vi "BCU参数读取-Auto.vi"(8 "CAN端口":u16(ring), 9 "设备索引号":u16(ring), 10 "CAN卡类型":u32(ring)=21, 11 "Myindex":dbl=1.0) -> (3 "成功":bool)   [LabVIEW 2013] (continued)
      n15 = property on="SOC(%)" class="DigNum (严格)"("Disabled"=w39) -> ()  [unwired: 2 in, 2 out]
      n16 = local write "等级 2"(T19."从板信息" ("等级 2")) -> ()
      n17 = local write "主板2"(T8."项目信息" ("主从板")) -> ()
      n18 = property class="MCListbox (严格)"(reference=w44, "ItemNames"=w40) -> ()  [unwired: 1 in, 2 out]
      n19 = property class="MCListbox (严格)"(reference=w43, "ItemNames"=w40) -> ()  [unwired: 1 in, 2 out]
      n20 = property class="MCListbox (严格)"(reference=w42, "ItemNames"=w40) -> ()  [unwired: 1 in, 2 out]
      n21 = property class="Bool (严格)"(reference=w61, "BoolText.TextColor"=u32 87470) -> ()  [unwired: 1 in, 2 out]
      n22 = property class="Bool (严格)"(reference=w62, "BoolText.TextColor"=w36) -> ()  [unwired: 1 in, 2 out]
      n23 = local write "主从板"(enum32{"单选选项2", "单选选项1"}."单选选项1" ("主从板")) -> ()
      n24 = property on="项目信息2" class="Clust (严格)"("DisabledEnum"=w39) -> ()  [unwired: 2 in, 2 out]
      n25 = property on="系统时钟" class="Str"("Disabled"=w39) -> ()  [unwired: 2 in, 2 out]
      n26 = property on="配置文件版本" class="Str"("Disabled"=w39) -> ()  [unwired: 2 in, 2 out]
      n27 = property on="车架(牌)号" class="Str"("Disabled"=w39) -> ()  [unwired: 2 in, 2 out]
      n28 = property on="产品编号" class="Str"("Disabled"=w39) -> ()  [unwired: 2 in, 2 out]
      n29 = property on="从板号" class="DigNum (严格)"("NumText.BGColor"=w36) -> ()  [unwired: 2 in, 2 out]
      n30 = property on="单选选项2 2" class="Bool (严格)"("BoolText.TextColor"=w36) -> ()  [unwired: 2 in, 2 out]
      n31 = local write "面板选择"(T7."读写参数" ("面板选择")) -> ()
      n32 = property on="单选选项1" class="Bool (严格)"("BoolText.TextColor"=u32 5898201) -> ()  [unwired: 2 in, 2 out]
      n33 = property on="单选选项2" class="Bool (严格)"("BoolText.TextColor"=w36) -> ()  [unwired: 2 in, 2 out]
      n34 = local write "主界面选项"(enum32{"单选选项1", "单选选项2", "单选选项2 2", "单选选项2 3"}."单选选项1" ("主界面选项")) -> ()
      n35 = local write "判定3"(w46) -> ()
      n36 = local write "清BUFF"(w46) -> ()
      n37 = local write "1"(w46) -> ()
      n38 = property on="从板个数" class="DigNum (严格)"("Visible"=w46) -> ()  [unwired: 2 in, 2 out]
      n39 = property on="从板个数" class="DigNum (严格)"("NumText.BGColor"=u32 16448250) -> ()  [unwired: 2 in, 2 out]
      n40 = Not(x=w46) -> (.not. x?=w65:bool)
      n41 = property on="主板选项" class="Tree (严格)"("Visible"=w46) -> ()  [unwired: 2 in, 2 out]
      n42 = property on="全部写入" class="Bool (严格)"("DisabledEnum"=2) -> ()  [unwired: 2 in, 2 out]
      n43 = property on="当前从板板号" class="DigNum (严格)"("Visible"=w65) -> ()  [unwired: 2 in, 2 out]
      n44 = property on="从板选项" class="Tree (严格)"("Visible"=w65) -> ()  [unwired: 2 in, 2 out]
      n45 = control-ref of="结果"() -> (w52:refnum<vi>)
      n46 = control-ref of="结果"() -> (w49:refnum<vi>)
      n47 = local write "强制停止版本读取"(w38) -> ()
      n48 = local write "强制终止读写标记"(w38) -> ()
      n49 = control-ref of="项目信息"() -> (w50:refnum<vi>)
      n50 = local write "判定2"(w38) -> ()
      n51 = local write "停止"(w38) -> ()
      n52 = local write "控制1"(w38) -> ()
      n53 = local write "消除"(w38) -> ()
      n54 = global write "EV05全局变量1.vi" "授权功能"(w38) -> ()
      n55 = local write "继电器超时处理"(w38) -> ()
      n56 = local write "1 6"(w38) -> ()
      n57 = local write "1 7"(w38) -> ()
      n58 = local write "1 8"(w38) -> ()
      n59 = local write "1 9"(w38) -> ()
      n60 = local write "1 10"(w38) -> ()
      n61 = local write "1 2"(w38) -> ()
      n62 = local write "1 3"(w38) -> ()
      n63 = local write "1 4"(w38) -> ()
      n64 = local write "1 5"(w38) -> ()
      n65 = local write "1 11"(w38) -> ()
      n66 = for {
        N: 100 -> [_]
        tunnel: w52 -> [w88]
        i -> [w86]
        n67 = Bundle(w86, 0) -> (w84:cluster{i32, i32})  [unwired: 1 out]
        n68 = property class="MCListbox (严格)"(reference=w88, "ActiveCell"=w84, "CellBG"=u32 16448250) -> ()  [unwired: 1 in, 2 out]
      }
      n69 = for {
        N: 100 -> [_]
        tunnel: w50 -> [w83]
        i -> [w82]
        n70 = Bundle(w82, 0) -> (w80:cluster{i32, i32})  [unwired: 1 out]
        n71 = property class="Tbl (严格)"(reference=w83, "Active Cell"=w80, "Cell BG Color"=u32 16448250) -> ()  [unwired: 1 in, 2 out]
      }
      n72 = for {
        N: 100 -> [_]
        tunnel: w49 -> [w93]
        i -> [w91]
        n73 = Bundle(w91, 0) -> (w89:cluster{i32, i32})  [unwired: 1 out]
        n74 = property class="MCListbox (严格)"(reference=w93, "ActiveCell"=w89, "CellBG"=u32 16448250) -> ()  [unwired: 1 in, 2 out]
      }
      n75 = stacked-sequence {
        tunnel: [_ w67] -> w45
        frame #0 {
          w66 = u32 21 items=["PCI5121"=1, "PCI9810"=2, "USBCAN1"=3, "USBCAN2"=4, "PCI9820"=5, "PCI5110"=7, "CANLite(mini)"=8, "ISA9620"=9, "ISA5420"=10, "PC104CAN"=11, "DNP9810"=13, "PCI9840B"=14, "PC104C2"=15, "PCI9820I"=16, "pec9920"=18, "USBCAN_E_U"=20, "USBCAN_2E_U"=21] ("CAN卡类型")
          n76 = local write "CAN卡类型"(w66) -> ()
        }
        frame #1 {
          w74 = u8 0 items=["Normal", "Listen Only"] ("工作方式")
          w73 = u8 1 items=["Dual Filter", "Single Filter"] ("滤波方式")
          n77 = local read "CAN卡类型"() -> (w68:u32)
          n78 = local read "设备索引号"() -> (w69:u16)
          n79 = local read "CAN端口"() -> (w70:u16)
          n80 = call "CAN_Init-8.6.vi"("CAN卡类型"=w68, "设备索引号"=w69, "CAN端口"=w70, "操作类型"=enum16{"初始化CAN", "关闭CAN"}."初始化CAN", "滤波方式"=w73, "Accept Code"=u32 3221225472, "簇"=T21 {"打开CAN"=TRUE, "初始化CAN"=TRUE, "开始CAN"=TRUE, "重启"=FALSE, "关闭CAN"=FALSE}, "Mask Code"=u32 1073741823 ("Accept Code"), "工作方式"=w74, "是否滤波"=TRUE, "滤波选择"=T20 {"fiter_mode"=1, "fiter_endid"=402653184, "fiter_startid"=419430399}) -> ("error out"=w67:errorcluster)  [unwired: 3 in, 5 out]
        }
      }
      n81 = local write "加热继电器(从)"(w38) -> ()
      n82 = local write "风机继电器(从)"(w38) -> ()
      n83 = local write "DO1"(w38) -> ()
      n84 = local write "DO2"(w38) -> ()
      n85 = local write "DO1 2"(w38) -> ()
      n86 = local write "正级继电器"(w38) -> ()
      n87 = local write "负级继电器"(w38) -> ()
      n88 = local write "加热继电器"(w38) -> ()
      n89 = local write "充电继电器"(w38) -> ()
      n90 = local write "风机继电器"(w38) -> ()
      n91 = local write "预充电继电器"(w38) -> ()
      n92 = property on="保存版本信息" class="Bool (严格)"("Visible"=w38) -> ()  [unwired: 2 in, 2 out]
      n93 = property on="单个读取" class="Bool (严格)"("Visible"=w38) -> ()  [unwired: 2 in, 2 out]
      n94 = property on="单个写入" class="Bool (严格)"("Visible"=w38) -> ()  [unwired: 2 in, 2 out]
      n95 = local write "正级继电器 12"(w38) -> ()
      n96 = local write "正级继电器 2"(w38) -> ()
      n97 = local write "正级继电器 3"(w38) -> ()
      n98 = local write "正级继电器 4"(w38) -> ()
      n99 = local write "正级继电器 5"(w38) -> ()
      n100 = local write "正级继电器 6"(w38) -> ()
      n101 = local write "正级继电器 7"(w38) -> ()
      n102 = local write "正级继电器 8"(w38) -> ()
      n103 = local write "正级继电器 9"(w38) -> ()
      n104 = local write "正级继电器 10"(w38) -> ()
      n105 = local write "正级继电器 11"(w38) -> ()
      n106 = property on="从板号" class="DigNum (严格)"("Visible"=w38) -> ()  [unwired: 2 in, 2 out]
      "电池故障" <- w40
      "模块版本值" <- w57
      "硬件版本" <- w58
      "模块版本名称" <- w57
      "平台软件版本" <- w58
      "项目软件版本" <- w58
      "模块个数" <- u8[] [0, 0, 0, 0, 0, 0, 0, 0, 0, 0, 0, 0, 0, 0, 0, 0, 0, 0, 0, 0, 0, 0, 0, 0, 0, 0, 0, 0, 0, 0, 0, 0] ("模块个数")
    }
  }
  n107 = stacked-sequence {
    tunnel: [w94] -> w24
    frame #0 {
      n108 = call <vilib>:"Set Busy.vi"() -> ()  [unwired: 10 in, 2 out]
      n109 = disable-structure shown="禁用" {
        frame Disabled {
          n110 = control-ref of="主板选项"() -> (w213:refnum<vi>)
          n111 = stacked-sequence {
            tunnel: w213 -> [w215 w373 w411]
            frame #0 {
              # "加热和充电控制参数"
              n112 = global read "功能码全局.vi" "主板控制类信息10"() -> (w225:bool[])
              n113 = Index Array(array=w225) -> (element #5=w219:bool, element #6=w217:bool, element #7=w218:bool, element #8=w216:bool)  [unwired: 8 in, 4 out]
              n114 = Not Or(1:w218, 2:w219) -> (0:w224:bool)
              n115 = Not Or(1:w216, 2:w217) -> (0:w222:bool)
              n116 = for {
                N: 8 -> [_]
                tunnel: w215 -> [w345]
                tunnel: w224 -> [w341]
                tunnel: [w340] -> w223
                i -> [w343]
                n117 = Add(x=w343, y=69) -> (x+y=w344:i32)
                n118 = property class="Tree (严格)"(reference=w345, "Active Item Row Number"=w344, "Disabled?"=w341) -> (error out=w340:errorcluster)  [unwired: 1 in, 1 out]
              }
              n119 = for {
                N: 9 -> [_]
                tunnel: w215 -> [w339]
                tunnel: w222 -> [w335]
                tunnel: w223 -> [w334]
                tunnel: [w333] -> w214
                i -> [w337]
                n120 = Add(x=w337, y=77) -> (x+y=w338:i32)
                n121 = property class="Tree (严格)"(reference=w339, error in=w334, "Active Item Row Number"=w338, "Disabled?"=w335) -> (error out=w333:errorcluster)  [unwired: 1 out]
              }
              n122 = stacked-sequence {
                tunnel: w215 -> [w245 _ _]
                tunnel: w214 -> [w244 _ _]
                frame #0 {
                  # "电池信息"
                  n123 = global read "功能码全局.vi" "主板版本号11"() -> (w246:bool[])
                  n124 = global read "功能码全局.vi" "主板项目信息4"() -> (w228:bool[])
                  n125 = Index Array(array=w246) -> (element #1=w242:bool, element #2=w241:bool, element #3=w235:bool, element #4=w229:bool, element #6=w234:bool, element #7=w233:bool, element #8=w232:bool)  [unwired: 8 in, 1 out]
                  n126 = Index Array(array=w228, index=4 ("索引")) -> (element=w226:bool)
                  n127 = Or(x=w235, y=w229) -> (x .or. y?=w230:bool)
                  n128 = Not(x=w233) -> (.not. x?=w237:bool)
                  n129 = Not(x=w232) -> (.not. x?=w236:bool)
                  n130 = Not(x=w234) -> (.not. x?=w238:bool)
                  n131 = property on="硬件版本号" class="Str"("Visible"=w235) -> ()  [unwired: 2 in, 2 out]
                  n132 = property on="读硬件版本号" class="Bool (严格)"("Visible"=w235) -> ()  [unwired: 2 in, 2 out]
                  n133 = property on="项目软件版本号" class="Str"("Visible"=w235) -> ()  [unwired: 2 in, 2 out]
                  n134 = property on="项目软本读取" class="Bool (严格)"("Visible"=w235) -> ()  [unwired: 2 in, 2 out]
                  n135 = property on="继电器屏1 2" class="TabCtl (严格)"("Visible"=w238) -> ()  [unwired: 2 in, 2 out]
                  n136 = property on="均衡屏" class="TabCtl (严格)"("Visible"=w236) -> ()  [unwired: 2 in, 2 out]
                  n137 = property on="继电器屏1 2" class="TabCtl (严格)"("Visible"=w238) -> ()  [unwired: 2 in, 2 out]
                  n138 = property on="DO屏" class="TabCtl (严格)"("Visible"=w237) -> ()  [unwired: 2 in, 2 out]
                  n139 = Compound Arithmetic op=OR(w234, w233, w232) -> (w231:bool)
                  n140 = Not Or(1:w241, 2:w242) -> (0:w240:bool)
                  n141 = stacked-sequence {
                    tunnel: w231 -> [_ w251 _]
                    tunnel: w230 -> [_ _ w255]
                    tunnel: w226 -> [w247 _ _]
                    frame #0 {
                      n142 = case shown="真" w247 {
                        frame False {
                        }
                        frame True {
                          n143 = local write "主界面选项"(enum32{"单选选项1", "单选选项2", "单选选项2 2", "单选选项2 3"}."单选选项2 3" ("主界面选项")) -> ()
                          n144 = local write "面板选择"(T7."高压板校正" ("面板选择")) -> ()
                        }
                      }
                      n145 = control-ref of="单选选项2 3"() -> (w248:refnum<vi>)
                      n146 = property class="Bool (严格)"(reference=w248, "Visible"=w247) -> ()  [unwired: 1 in, 2 out]
                    }
                    frame #1 {
                      n147 = control-ref of="单选选项2 2"() -> (w252:refnum<vi>)
                      n148 = case shown="真" w251 {
                        frame False {
                        }
                        frame True {
                          n149 = local write "主界面选项"(enum32{"单选选项1", "单选选项2", "单选选项2 2", "单选选项2 3"}."单选选项2 2" ("主界面选项")) -> ()
                          n150 = local write "面板选择"(enum32{"读写参数", "版本读取", "其它诊断"}."其它诊断" ("选项卡控件 2")) -> ()
                        }
                      }
                      n151 = property class="Bool (严格)"(reference=w252, "Visible"=w251) -> ()  [unwired: 1 in, 2 out]
                    }
                    frame #2 {
                      n152 = control-ref of="单选选项2"() -> (w256:refnum<vi>)
                      n153 = case shown="真" w255 {
                        frame False {
                        }
                        frame True {
                          n154 = local write "主界面选项"(enum32{"单选选项1", "单选选项2", "单选选项2 2", "单选选项2 3"}."单选选项2" ("主界面选项")) -> ()
                          n155 = local write "面板选择"(enum32{"读写参数", "版本读取", "其它诊断"}."版本读取" ("选项卡控件 2")) -> ()
                        }
                      }
                      n156 = property class="Bool (严格)"(reference=w256, "Visible"=w255) -> ()  [unwired: 1 in, 2 out]
                    }
                  }
                  n157 = for {
                    N: 5 -> [_]
                    tunnel: w245 -> [w265]
                    tunnel: w240 -> [w261]
                    tunnel: w244 -> [w260]
                    tunnel: [w259] -> w243
                    i -> [w263]
                    n158 = Add(x=w263, y=86) -> (x+y=w264:i32)
                    n159 = property class="Tree (严格)"(reference=w265, error in=w260, "Active Item Row Number"=w264, "Disabled?"=w261) -> (error out=w259:errorcluster)  [unwired: 1 out]
                  }
                  n160 = property on="模块软件版本 2" class="MCListbox (严格)"("Visible"=w229) -> ()  [unwired: 2 in, 2 out]
                  n161 = property on="模块软件版本" class="Enum (严格)"("Visible"=w229) -> ()  [unwired: 2 in, 2 out]
                  n162 = property on="平台软件版本号" class="Str"("Visible"=w229) -> ()  [unwired: 2 in, 2 out]
                  n163 = property on="模块版本读取" class="Bool (严格)"("Visible"=w229) -> ()  [unwired: 2 in, 2 out]
                  n164 = property on="平台软件版本读取" class="Bool (严格)"("Visible"=w229) -> ()  [unwired: 2 in, 2 out]
                  n165 = call <vilib>:"Clear Errors.vi"("error in (no error)"=w243) -> ()  [unwired: 6 in, 1 out]
                }
                frame #1 {
                  n166 = global read "功能码全局.vi" "主板项目信息7"() -> (w305:bool[])
                  n167 = global read "功能码全局.vi" "主板控制类信息10"() -> (w301:bool[])
                  n168 = global read "功能码全局.vi" "主板故障阀值9"() -> (w304:bool[])
                  n169 = global read "功能码全局.vi" "主板项目信息4"() -> (w283:bool[])
                  n170 = global read "功能码全局.vi" "主板项目信息5"() -> (w292:bool[])
                  n171 = global read "功能码全局.vi" "主板项目信息6"() -> (w282:bool[])
                  n172 = global read "功能码全局.vi" "主板版本号11"() -> (w291:bool[])
                  n173 = Delete From Array(array=w282, length=1 ("长度"), index=0 ("索引")) -> (deleted portion=w293:bool[], array with subset deleted=w309:bool[])
                  n174 = Index Array(array=w283, index #1=5 ("索引"), index #2=6 ("索引"), index #3=7 ("索引")) -> (element #1=w294:bool, element #2=w310:bool, element #3=w266:bool)
                  n175 = Index Array(array=w291) -> (element #1=w298:bool, element #2=w314:bool)  [unwired: 2 in]
                  n176 = Array Subset(array=w304, index=2 ("索引"), length=3 ("长度")) -> (w296:bool[])
                  n177 = Delete From Array(array=w305, length=3 ("索引"), index=2 ("长度")) -> (deleted portion=w295:bool[], array with subset deleted=w311:bool[])
                  n178 = Array Subset(array=w301, index=4 ("索引"), length=2 ("长度")) -> (w297:bool[])
                  n179 = global read "功能码全局.vi" "18"() -> (w274:bool[])
                  n180 = global read "功能码全局.vi" "16"() -> (w275:bool[])
                  n181 = Insert Into Array(array=w292, new element #1=w293, new element #2=w294, new element #3=w295, new element #4=w296, new element #5=w297, new element #6=w298) -> (w315:bool[])  [unwired: 1 in]
                  n182 = Array Subset(array=w301, index=6 ("索引"), length=2 ("长度")) -> (w313:bool[])
                  n183 = Array Subset(array=w304, index=5 ("索引"), length=3 ("长度")) -> (w312:bool[])
                  n184 = And Array Elements(Boolean array=w315) -> (logical AND=w280:bool)
                  n185 = Array Subset(array=w274, index=0 ("索引"), length=8 ("长度")) -> (w272:bool[])
                  n186 = Array Subset(array=w275, index=4 ("索引"), length=4 ("长度")) -> (w271:bool[])
                  n187 = Or Array Elements(Boolean array=w315) -> (logical OR=w267:bool)
                  n188 = Insert Into Array(array=w309, new element #1=w310, new element #2=w311, new element #3=w312, new element #4=w313, new element #5=w314) -> (w316:bool[])  [unwired: 1 in]
                  n189 = property on="全部读取" class="Bool (严格)"("Visible"=w280) -> ()  [unwired: 2 in, 2 out]
                  n190 = global read "功能码全局.vi" "15"() -> (w273:bool[])
                  n191 = And Array Elements(Boolean array=w316) -> (logical AND=w281:bool)
                  n192 = property on="全部写入" class="Bool (严格)"("Visible"=w281) -> ()  [unwired: 2 in, 2 out]
                  n193 = Or Array Elements(Boolean array=w316) -> (logical OR=w317:bool)
                  n194 = Insert Into Array(array=w273, new element #1=w272, new element #2=w271) -> (w270:bool[])  [unwired: 1 in]
                  n195 = Or Array Elements(Boolean array=w270) -> (logical OR=w269:bool)
                  n196 = Compound Arithmetic op=OR(w266, w267, w317, w269) -> (w318:bool)
                  n197 = case shown="真" w318 {
                    frame False {
                    }
                    frame True {
                      n198 = local write "主界面选项"(enum32{"单选选项1", "单选选项2", "单选选项2 2", "单选选项2 3"}."单选选项1" ("主界面选项")) -> ()
                      n199 = local write "面板选择"(enum32{"读写参数", "版本读取", "其它诊断"}."读写参数" ("选项卡控件 2")) -> ()
                    }
                  }
                  n200 = property on="单选选项1" class="Bool (严格)"("Visible"=w318) -> ()  [unwired: 2 in, 2 out]
                }
                frame #2 {
                  n201 = control-ref of="单选选项2 2"() -> (w325:refnum<vi>)
                  n202 = control-ref of="单选选项2 3"() -> (w321:refnum<vi>)
                  n203 = control-ref of="单选选项2"() -> (w327:refnum<vi>)
                  n204 = control-ref of="单选选项1"() -> (w326:refnum<vi>)
                  n205 = local read "主界面选项"() -> (w330:enum32{"单选选项1", "单选选项2", "单选选项2 2", "单选选项2 3"})
                  n206 = Build Array(w326, w327, w325, w321) -> (w324:refnum<vi>[])
                  n207 = Delete From Array(array=w324, index=w330) -> (deleted portion=w328:refnum<vi>, array with subset deleted=w329:refnum<vi>[])  [unwired: 1 in]
                  n208 = property class="Bool (严格)"(reference=w328, "BoolText.TextColor"=u32 87470) -> ()  [unwired: 1 in, 2 out]
                  n209 = for {
                    tunnel: u32 16777215 -> [w332]
                    tunnel: w329 -> [w331] mode=indexing
                    n210 = property class="Bool (严格)"(reference=w331, "BoolText.TextColor"=w332) -> ()  [unwired: 1 in, 2 out]
                  }
                }
              }
            }
            frame #1 {
              # "项目信息"
              # "SOC"
              # "SOH"
              # "电池额定实际容量"
              # "车牌号"
              # "产品编号"
              # "电压个数"
              # "通道电压数"
              # "温度个数"
              # "电压起始值"
              # "温度起始值"
              # "配置文件版本"
              # "系统时钟"
              # "校正时钟"
              n211 = global read "功能码全局.vi" "主板项目信息5"() -> (w406:bool[])
              n212 = global read "功能码全局.vi" "主板项目信息6"() -> (w405:bool[])
              n213 = global read "功能码全局.vi" "主板项目信息7"() -> (w382:bool[])
              n214 = global read "功能码全局.vi" "主板项目信息4"() -> (w353:bool[])
              n215 = Index Array(array=w406) -> (element #1=w403:bool, element #2=w400:bool, element #3=w397:bool, element #4=w394:bool, element #5=w390:bool, element #6=w388:bool, element #7=w385:bool, element #8=w381:bool)  [unwired: 8 in]
              n216 = Index Array(array=w405) -> (element #1=w378:bool, element #2=w402:bool, element #3=w399:bool, element #4=w396:bool, element #5=w393:bool, element #6=w389:bool, element #7=w387:bool, element #8=w384:bool)  [unwired: 8 in]
              n217 = Index Array(array=w382) -> (element #1=w380:bool, element #2=w377:bool, element #3=w375:bool, element #4=w370:bool, element #5=w367:bool, element #6=w374:bool, element #7=w368:bool, element #8=w366:bool)  [unwired: 8 in]
              n218 = Index Array(array=w353) -> (element #6=w349:bool, element #7=w348:bool, element #8=w352:bool)  [unwired: 8 in, 5 out]
              n219 = Not(x=w352) -> (.not. x?=w351:bool)
              n220 = Not Or(1:w348, 2:w349) -> (0:w347:bool)
              n221 = Not Or(1:w402, 2:w403) -> (0:w365:bool)
              n222 = Not Or(1:w399, 2:w400) -> (0:w364:bool)
              n223 = Not Or(1:w396, 2:w397) -> (0:w363:bool)
              n224 = Not Or(1:w393, 2:w394) -> (0:w362:bool)
              n225 = Not Or(1:w389, 2:w390) -> (0:w361:bool)
              n226 = Not Or(1:w387, 2:w388) -> (0:w360:bool)
              n227 = Not Or(1:w384, 2:w385) -> (0:w359:bool)
              n228 = Not Or(1:w380, 2:w381) -> (0:w358:bool)
              n229 = Not Or(1:w374, 2:w375) -> (0:w356:bool)
              n230 = Not Or(1:w366, 2:w367) -> (0:w354:bool)
              n231 = Not Or(1:w368, 2:w370) -> (0:w355:bool)
              n232 = Not Or(1:w377, 2:w378) -> (0:w357:bool)
              n233 = Compound Arithmetic op=OR(w351, w365, w364, w363, w362, w361, w360, w359, w358, w357, w356, w355, w354) -> (w346:bool)
              "项目信息结果" <- w346
              n234 = property class="Tree (严格)"(reference=w373, "Active Item Row Number"=9 ("活动项:行数"), "Disabled?"=w347, "Active Item Row Number"=1 ("活动项:行数"), "Disabled?"=w346, "Active Item Row Number"=0 ("活动项:行数"), "Disabled?"=w351, "Active Item Row Number"=3 ("活动项:行数"), "Disabled?"=w365, "Active Item Row Number"=4 ("活动项:行数"), "Disabled?"=w364, "Active Item Row Number"=5 ("活动项:行数"), "Disabled?"=w363, "Active Item Row Number"=6 ("活动项:行数"), "Disabled?"=w362, "Active Item Row Number"=7 ("活动项:行数"), "Disabled?"=w361, "Active Item Row Number"=8 ("活动项:行数"), "Disabled?"=w360, "Active Item Row Number"=11 ("活动项:行数"), "Disabled?"=w359, "Active Item Row Number"=12 ("活动项:行数"), "Disabled?"=w358, "Active Item Row Number"=13 ("活动项:行数"), "Disabled?"=w357, "Active Item Row Number"=2 ("活动项:行数"), "Disabled?"=w356, "Active Item Row Number"=10 ("活动项:行数"), "Disabled?"=w355, "Active Item Row Number"=14 ("活动项:行数"), "Disabled?"=w354) -> ()  [unwired: 1 in, 2 out]
            }
            frame #2 {
              w416 = 18
              # "一二三级故障"
              n235 = global read "功能码全局.vi" "主板故障阀值9"() -> (w422:bool[])
              n236 = Index Array(array=w422) -> (element #3=w421:bool, element #4=w418:bool, element #5=w415:bool, element #6=w420:bool, element #7=w417:bool, element #8=w414:bool)  [unwired: 8 in, 2 out]
              n237 = Not Or(1:w420, 2:w421) -> (0:w410:bool)
              n238 = Not Or(1:w417, 2:w418) -> (0:w408:bool)
              n239 = Not Or(1:w414, 2:w415) -> (0:w409:bool)
              n240 = for {
                N: w416 -> [_]
                tunnel: w411 -> [w442]
                tunnel: w410 -> [w438]
                tunnel: [w437] -> w419
                i -> [w440]
                n241 = Add(x=w440, y=15) -> (x+y=w441:i32)
                n242 = property class="Tree (严格)"(reference=w442, "Active Item Row Number"=w441, "Disabled?"=w438) -> (error out=w437:errorcluster)  [unwired: 1 in, 1 out]
              }
              n243 = for {
                N: w416 -> [_]
                tunnel: w411 -> [w436]
                tunnel: w408 -> [w432]
                tunnel: w419 -> [w431]
                tunnel: [w430] -> w413
                i -> [w434]
                n244 = Add(x=w434, y=33) -> (x+y=w435:i32)
                n245 = property class="Tree (严格)"(reference=w436, error in=w431, "Active Item Row Number"=w435, "Disabled?"=w432) -> (error out=w430:errorcluster)  [unwired: 1 out]
              }
              n246 = for {
                N: w416 -> [_]
                tunnel: w411 -> [w429]
                tunnel: w409 -> [w425]
                tunnel: w413 -> [w424]
                tunnel: [w423] -> w412
                i -> [w427]
                n247 = Add(x=w427, y=51) -> (x+y=w428:i32)
                n248 = property class="Tree (严格)"(reference=w429, error in=w424, "Active Item Row Number"=w428, "Disabled?"=w425) -> (error out=w423:errorcluster)  [unwired: 1 out]
              }
              n249 = call <vilib>:"Clear Errors.vi"("error in (no error)"=w412) -> ()  [unwired: 6 in, 1 out]
            }
          }
        }
        frame Enabled {
        }
      }
      n250 = disable-structure shown="禁用" {
        disable-tunnel: [w95 _] -> w94
        frame Disabled {
          n251 = control-ref of="从板选项"() -> (w96:refnum<vi>)
          n252 = stacked-sequence {
            tunnel: w96 -> [w99 w136 w178]
            tunnel: [w97 _ _] -> w95
            frame #0 {
              n253 = global read "功能码全局.vi" "15"() -> (w122:bool[])
              n254 = global read "功能码全局.vi" "16"() -> (w113:bool[])
              n255 = Index Array(array=w122) -> (element #1=w121:bool, element #2=w119:bool, element #3=w117:bool, element #4=w115:bool, element #5=w120:bool, element #6=w118:bool, element #7=w116:bool, element #8=w114:bool)  [unwired: 8 in]
              n256 = Index Array(array=w113) -> (element #5=w104:bool, element #6=w112:bool, element #7=w103:bool, element #8=w111:bool)  [unwired: 8 in, 4 out]
              n257 = Not Or(1:w111, 2:w112) -> (0:w101:bool)
              n258 = Not Or(1:w103, 2:w104) -> (0:w102:bool)
              n259 = Not Or(1:w120, 2:w121) -> (0:w107:bool)
              n260 = Not Or(1:w118, 2:w119) -> (0:w108:bool)
              n261 = Not Or(1:w116, 2:w117) -> (0:w109:bool)
              n262 = Not Or(1:w114, 2:w115) -> (0:w110:bool)
              n263 = Compound Arithmetic op=OR(w107, w108, w109, w110, w101) -> (w106:bool)
              "从板项目信息" <- w106
              n264 = property class="Tree (严格)"(reference=w99, "Active Item Row Number"=1 ("活动项:行数"), "Disabled?"=w106, "Active Item Row Number"=2 ("活动项:行数"), "Disabled?"=w107, "Active Item Row Number"=3 ("活动项:行数"), "Disabled?"=w108, "Active Item Row Number"=4 ("活动项:行数"), "Disabled?"=w109, "Active Item Row Number"=5 ("活动项:行数"), "Disabled?"=w110, "Active Item Row Number"=0 ("活动项:行数"), "Disabled?"=w102) -> (error out=w98:errorcluster)  [unwired: 1 in, 1 out]
              n265 = for {
                N: 8 -> [_]
                tunnel: w99 -> [w134]
                tunnel: w101 -> [w130]
                tunnel: w98 -> [w129]
                tunnel: [w128] -> w97
                i -> [w132]
                n266 = Add(x=w132, y=6) -> (x+y=w133:i32)
                n267 = property class="Tree (严格)"(reference=w134, error in=w129, "Active Item Row Number"=w133, "Disabled?"=w130) -> (error out=w128:errorcluster)  [unwired: 1 out]
              }
              n268 = call <vilib>:"Clear Errors.vi"("error in (no error)"=w97) -> ()  [unwired: 6 in, 1 out]
            }
            frame #1 {
              w147 = 8
              n269 = global read "功能码全局.vi" "18"() -> (w156:bool[])
              n270 = Index Array(array=w156) -> (element #1=w139:bool, element #2=w140:bool, element #3=w155:bool, element #4=w150:bool, element #5=w144:bool, element #6=w154:bool, element #7=w149:bool, element #8=w143:bool)  [unwired: 8 in]
              n271 = Not Or(1:w140, 2:w139) -> (0:w135:bool)
              n272 = property class="Tree (严格)"(reference=w136, "Active Item Row Number"=46 ("活动项:行数"), "Disabled?"=w135, "Active Item Row Number"=47 ("活动项:行数"), "Disabled?"=w135, "Active Item Row Number"=48 ("活动项:行数"), "Disabled?"=w135) -> ()  [unwired: 1 in, 2 out]
              n273 = Not Or(1:w143, 2:w144) -> (0:w142:bool)
              n274 = Not Or(1:w154, 2:w155) -> (0:w153:bool)
              n275 = Not Or(1:w149, 2:w150) -> (0:w148:bool)
              n276 = for {
                N: w147 -> [_]
                tunnel: w136 -> [w177]
                tunnel: w153 -> [w173]
                tunnel: "error out" -> [w172]
                tunnel: [w171] -> w151
                i -> [w175]
                n277 = Add(x=w175, y=14) -> (x+y=w176:i32)
                n278 = property class="Tree (严格)"(reference=w177, error in=w172, "Active Item Row Number"=w176, "Disabled?"=w173) -> (error out=w171:errorcluster)  [unwired: 1 out]
              }
              n279 = for {
                N: w147 -> [_]
                tunnel: w136 -> [w170]
                tunnel: w148 -> [w166]
                tunnel: w151 -> [w165]
                tunnel: [w164] -> w146
                i -> [w168]
                n280 = Add(x=w168, y=22) -> (x+y=w169:i32)
                n281 = property class="Tree (严格)"(reference=w170, error in=w165, "Active Item Row Number"=w169, "Disabled?"=w166) -> (error out=w164:errorcluster)  [unwired: 1 out]
              }
              n282 = for {
                N: w147 -> [_]
                tunnel: w136 -> [w163]
                tunnel: w142 -> [w159]
                tunnel: w146 -> [w158]
                tunnel: [w157] -> w145
                i -> [w161]
                n283 = Add(x=w161, y=30) -> (x+y=w162:i32)
                n284 = property class="Tree (严格)"(reference=w163, error in=w158, "Active Item Row Number"=w162, "Disabled?"=w159) -> (error out=w157:errorcluster)  [unwired: 1 out]
              }
              n285 = call <vilib>:"Clear Errors.vi"("error in (no error)"=w145) -> ()  [unwired: 6 in, 1 out]
            }
            frame #2 {
              n286 = global read "功能码全局.vi" "23"() -> (w202:bool[])
              n287 = global read "功能码全局.vi" "24"() -> (w200:bool[])
              n288 = Index Array(array=w202) -> (element #3=w201:bool, element #4=w198:bool, element #5=w196:bool, element #6=w194:bool, element #7=w192:bool, element #8=w190:bool)  [unwired: 8 in, 2 out]
              n289 = Index Array(array=w200) -> (element #3=w199:bool, element #4=w197:bool, element #5=w195:bool, element #6=w193:bool, element #7=w191:bool, element #8=w189:bool)  [unwired: 8 in, 2 out]
              n290 = Not Or(1:w199, 2:w201) -> (0:w188:bool)
              n291 = Not Or(1:w197, 2:w198) -> (0:w183:bool)
              n292 = Not Or(1:w195, 2:w196) -> (0:w184:bool)
              n293 = Not Or(1:w193, 2:w194) -> (0:w185:bool)
              n294 = Not Or(1:w191, 2:w192) -> (0:w187:bool)
              n295 = Not Or(1:w189, 2:w190) -> (0:w186:bool)
              n296 = Build Array(w188, w188, w187, w186, w185, w184, w183) -> (w181:bool[])
              n297 = And Array Elements(Boolean array=w181) -> (logical AND=w182:bool)
              n298 = Insert Into Array(array=w181, index=0 ("索引"), new element=w182) -> (w179:bool[])
              n299 = for {
                N: 8 -> [_]
                tunnel: w178 -> [w212]
                tunnel: w179 -> [w208] mode=indexing
                tunnel: errorcluster {"status"=FALSE, "code"=0, "source"=""} ("error out 2") -> [w207]
                tunnel: [w206] -> w204
                i -> [w210]
                n300 = Add(x=w210, y=38) -> (x+y=w211:i32)
                n301 = property class="Tree (严格)"(reference=w212, error in=w207, "Active Item Row Number"=w211, "Disabled?"=w208) -> (error out=w206:errorcluster)  [unwired: 1 out]
              }
              n302 = call <vilib>:"Clear Errors.vi"("error in (no error)"=w204) -> ()  [unwired: 6 in, 1 out]
            }
          }
        }
        frame Enabled {
        }
      }
    }
  }
  n303 = Index Array(array=w14, index (col)=0 ("索引 (行)")) -> (element=w17:string[])  [unwired: 1 in]
  n304 = Index Array(array=w14, index (col)=1 ("禁用的索引 (列)")) -> (element=w7:string[])  [unwired: 1 in]
  n305 = local read "从板个数"() -> (w9:dbl)
  n306 = Array Subset(array=w17, index=0 ("索引"), length=w9) -> (w16:string[])
  n307 = Array Subset(array=w17, index=10 ("索引"), length=w9) -> (w15:string[])
  n308 = Array Subset(array=w7, index=0 ("索引"), length=w9) -> (w13:string[])
  n309 = Array Subset(array=w7, index=10 ("索引"), length=w9) -> (w8:string[])
  n310 = Insert Into Array(array=w16, new element=w15) -> (w6:string[])  [unwired: 1 in]
  n311 = Insert Into Array(array=w13, new element=w8) -> (w5:string[])  [unwired: 1 in]
  n312 = Build Array(w6, w5) -> (w4:string[][])
  n313 = local write "停止"(FALSE ("停止")) -> ()
  n314 = local write "项目信息 2"(string[][] [["电压个数", "36"], ["温度个数", "45"], ["第一个保险通道", "0"], ["第一个保险位置", "0"], ["第二个保险通道", "0"], ["第二个保险位置", "0"], ["第三个保险通道", "0"], ["第三个保险位置", "0"], ["第四个保险通道", "0"], ["第四个保险位置", "0"], ["第五个保险通道", "0"], ["第五个保险位置", "0"], ["第六个保险通道", "0"], ["第六个保险位置", "0"], ["第七个保险通道", "0"], ["第七个保险位置", "0"], ["第八个保险通道", "0"], ["第八个保险位置", "0"], ["第九个保险通道", "0"], ["第九个保险位置", "0"], ["第十个保险通道", "0"], ["第十个保险位置", "0"], ["第1通道电压个数", "11"], ["第2通道电压个数", "12"], ["第3通道电压个数", "12"], ["第4通道电压个数", "12"], ["第5通道电压个数", "12"]] ("项目信息 2")) -> ()
  n315 = Transpose 2D Array(2D array=w4) -> (transposed array=w3:string[][])
  n316 = local write "项目信息"(w3) -> ()
  n317 = stacked-sequence {
    tunnel: w21 -> [_]
    tunnel: w24 -> [_]
    frame #0 {
      n318 = call <vilib>:"Unset Busy.vi"() -> ()  [unwired: 11 in, 1 out]
    }
  }
  n319 = Obtain Queue(name (unnamed)=w33, element data type=w33, error in (no error)=w21) -> (queue out=w32:refnum<queue>, error out=w1:errorcluster)  [unwired: 2 in, 1 out]
  n320 = Obtain Queue(element data type="读参数") -> (queue out=w26:refnum<queue>, error out=w25:errorcluster)  [unwired: 4 in, 1 out]
  n321 = case shown="无错误" w1 {
    selector: w1 -> [w443 _]
    frame No Error {
      n322 = case shown="\"全部读取\"" "全部读取" {
        tunnel: w443 -> [_ _ _ _ w1084 _ _ _ _ _ _ _ _ _ _]
        frame "假", Default {
          n323 = local write "强制终止读写标记"(FALSE ("强制终止读写标记")) -> ()
        }
        frame "单个写入" {
          n324 = local read "主从选择"() -> (w454:enum32{"主板", "从板"})
          n325 = case shown="\"从板\"" w454 {
            tunnel: [w465 w480] -> w451
            tunnel: [0.0 w478] -> w455
            tunnel: [_ w479] -> w453
            tunnel: [w463 _] -> w452
            frame "主板", Default {
              n326 = flat-sequence {
                tunnel: [w477] -> w463
                frame #0 {
                  n327 = control-ref of="高压参数"() -> (w468:refnum<vi>)
                  n328 = control-ref of="电池信息"() -> (w469:refnum<vi>)
                  n329 = control-ref of="一级故障"() -> (w475:refnum<vi>)
                  n330 = control-ref of="一级故障 2"() -> (w473:refnum<vi>)
                  n331 = control-ref of="一级故障 3"() -> (w472:refnum<vi>)
                  n332 = control-ref of="加热控制参数"() -> (w471:refnum<vi>)
                  n333 = control-ref of="充电控制参数"() -> (w470:refnum<vi>)
                  n334 = control-ref of="项目信息"() -> (w474:refnum<vi>)
                  n335 = control-ref of="项目信息2"() -> (w476:refnum<vi>)
                  n336 = local read "主板数据"() -> (w466:T4)
                  n337 = Bundle(cluster=w466, "项目信息"=w474, "一级故障 4"=w476, "一级故障"=w475, "一级故障 2"=w473, "一级故障 3"=w472, "加热控制参数"=w471, "充电控制参数"=w470, "高压参数"=w468, "电池信息"=w469) -> (w467:T4)
                  n338 = local write "主板数据"(w467) -> ()
                }
                frame #1 {
                  n339 = control-ref of="主板数据"() -> (w477:refnum<vi>)
                }
              }
              n340 = local read "主板选项"() -> (w465:string)
            }
            frame "从板" {
              n341 = stacked-sequence {
                tunnel: [_ w491] -> w479
                frame #0 {
                  n342 = control-ref of="从板号"() -> (w490:refnum<vi>)
                  n343 = control-ref of="项目信息 2"() -> (w489:refnum<vi>)
                  n344 = control-ref of="均衡参数"() -> (w484:refnum<vi>)
                  n345 = control-ref of="加热控制参数"() -> (w488:refnum<vi>)
                  n346 = control-ref of="一级故障(从板)"() -> (w487:refnum<vi>)
                  n347 = control-ref of="二级故障(从板)"() -> (w486:refnum<vi>)
                  n348 = control-ref of="三级故障(从板)"() -> (w485:refnum<vi>)
                  n349 = control-ref of="电池组信息"() -> (w481:refnum<vi>)
                  n350 = local read "从板信息"() -> (w482:T2)
                  n351 = Bundle(cluster=w482, "从板号"=w490, "项目信息 2"=w489, "加热控制参数"=w488, "一级故障(从板)"=w487, "二级故障(从板)"=w486, "三级故障(从板)"=w485, "电池组信息(从板)"=w481, "均衡参数"=w484) -> (w483:T2)
                  n352 = local write "从板信息"(w483) -> ()
                }
                frame #1 {
                  n353 = control-ref of="从板信息"() -> (w491:refnum<vi>)
                }
              }
              n354 = local read "从板选项"() -> (w480:string)
              n355 = local read "从板号"() -> (w478:u8)
            }
          }
          n356 = local read "从板个数"() -> (w456:dbl)
          n357 = local read "二维码信息 2"() -> (w446:string)
          n358 = local read "二维码信息"() -> (w447:string)
          n359 = local read "快换"() -> (w457:bool)
          n360 = call "输入数据解析.vi"("单个参数补充"=w456, "从板号"=w455, "主板二维码"=w447, "从板二维码"=w446, "主板引用"=w452, "从板引用"=w453, "主板选项"=w451, "枚举"=w454, "快换"=w457) -> ("输出数组"=w461:dbl[][], "数组长度"=w460:dbl[], "循环次数"=w450:i32, "命令"=w459:u32, "名称"=w449:string[], "命令序号"=w458:u32[])  [unwired: 1 out]
          n361 = for {
            N: w450 -> [w497]
            tunnel: w461 -> [w507]
            tunnel: w460 -> [w506]
            tunnel: w459 -> [w505]
            tunnel: w458 -> [w504]
            tunnel: w455 -> [w495]
            tunnel: w451 -> [w503]
            tunnel: w449 -> [w499]
            tunnel: [w492] -> w448
            i -> [w498]
            n362 = Index Array(array=w507, index (row)=w498) -> (element=w502:dbl[])  [unwired: 1 in]
            n363 = Index Array(array=w506, index=w498) -> (element=w501:dbl)
            n364 = Index Array(array=w499, index=w498) -> (element=w496:string)
            n365 = case shown="\"假\", 默认" w496 {
              tunnel: [w509 w510] -> w494
              tunnel: w495 -> [w509 _]
              tunnel: [TRUE ("确定") w511] -> w493
              frame "假", Default {
              }
              frame "从板号" {
                n366 = call "请输入当前从板板号"() -> ("当前从板板号"=w510:dbl, "确定"=w511:bool)  [unwired: 17 in, 1 out]
                n367 = local write "当前从板板号"(w510) -> ()
              }
            }
            n368 = Index Array(array=w504, index=w498) -> (element=w500:u32)
            n369 = global write "全局 1.vi" "名称"(w496) -> ()
            n370 = case shown="真" w493 {
              tunnel: w505 -> [_ w521]
              tunnel: w503 -> [_ w520]
              tunnel: w502 -> [_ w519]
              tunnel: w501 -> [_ w518]
              tunnel: w500 -> [_ w517]
              tunnel: w498 -> [_ w516]
              tunnel: w496 -> [_ w515]
              tunnel: w497 -> [_ w514]
              tunnel: w494 -> [_ w513]
              tunnel: [_ w512] -> w492
              frame False {
                n371 = call <vilib>:"Unset Busy.vi"() -> ()  [unwired: 11 in, 1 out]
              }
              frame True {
                n372 = stacked-sequence {
                  seq-local: [_ _ _ w549 _ _] -> [_ _ _ _ w558 _]
                  tunnel: w519 -> [_ _ w534 _ _ _]
                  tunnel: w518 -> [_ _ w533 _ _ _]
                  tunnel: w521 -> [_ _ w527 _ _ _]
                  tunnel: w517 -> [_ _ w525 _ _ _]
                  tunnel: w520 -> [_ _ _ _ _ _]
                  tunnel: w516 -> [_ _ _ _ _ w569]
                  tunnel: w515 -> [_ _ _ _ w557 _]
                  tunnel: w514 -> [_ _ _ _ _ w570]
                  tunnel: w513 -> [_ _ w526 _ _ _]
                  tunnel: [_ _ _ _ _ w567] -> w512
                  frame #0 {
                    w523 = FALSE ("流控帧")
                    w522 = TRUE ("流控帧 2")
                    n373 = call <vilib>:"Set Busy.vi"("disable click? (T)"=w523) -> ()  [unwired: 3 in, 8 out]
                    n374 = global write "EV05全局变量1.vi" "读取超时"(w523) -> ()
                    n375 = global write "EV05全局变量1.vi" "流控帧"(w523) -> ()
                    n376 = local write "消除"(w522) -> ()
                    n377 = local write "控制1"(w522) -> ()
                    n378 = global write "EV05全局变量1.vi" "流控帧 2"(w522) -> ()
                    n379 = local write "写?"(w522) -> ()
                  }
                  frame #1 {
                    n380 = Wait Until Next ms Multiple(millisecond multiple=u32 50 ("毫秒倍数")) -> ()  [unwired: 1 out]
                  }
                  frame #2 {
                    n381 = local read "设备索引号"() -> (w529:u16)
                    n382 = local read "CAN卡类型"() -> (w530:u32)
                    n383 = Increment(x=w533) -> (x+1=w532:dbl)
                    n384 = local read "CAN端口"() -> (w528:u16)
                    n385 = local write "命令"(w527) -> ()
                    n386 = local write "命令序号"(w525) -> ()
                    n387 = Reshape Array(w534, w532) -> (w531:dbl[])
                    n388 = stacked-sequence {
                      tunnel: w531 -> [_ w548]
                      tunnel: w530 -> [w537 w547]
                      tunnel: w529 -> [w536 w546]
                      tunnel: w528 -> [w535 w545]
                      tunnel: w527 -> [_ w544]
                      tunnel: w526 -> [_ w543]
                      tunnel: w525 -> [_ w542]
                      frame #0 {
                        n389 = disable-structure shown="禁用" {
                          disable-tunnel: w537 -> [w540 _]
                          disable-tunnel: w536 -> [w539 _]
                          disable-tunnel: w535 -> [w538 _]
                          frame Disabled {
                            n390 = dll-call lib="PTH1abs FBluewave New EnergySVN_WorkAutoTest_TestStandtrunkAutoTest_TestStandDriverZlgCanBHN01è¯»ååæ°data\nkerneldlls\nusbcan.dll" fn="VCI_ClearBuffer"("DeviceType"=w540, "DeviceInd"=w539, "CANInd"=w538) -> (error out=w541:errorcluster)  [unwired: 4 in, 4 out]
                            n391 = call <vilib>:"Clear Errors.vi"("error in (no error)"=w541) -> ()  [unwired: 6 in, 1 out]
                          }
                          frame Enabled {
                          }
                        }
                      }
                      frame #1 {
                        n392 = call "多帧发送机制(EV05).vi"("can卡类型"=w547, "设备索引号"=w546, "CAN端口"=w545, "命令"=w544, "板号"=w543, "命令序号"=w542, "输入数据"=w548) -> ()  [unwired: 2 in, 11 out]
                      }
                    }
                  }
                  frame #3 {
                    n393 = while {
                      tunnel: [w551] -> w549
                      i -> [w555]
                      stop <- w552 stop-if-true
                      n394 = local read "强制终止读写标记"() -> (w550:bool)
                      n395 = global read "EV05全局变量1.vi" "读取超时"() -> (w551:bool)
                      n396 = Greater Or Equal?(x=w555, y=30) -> (x >= y?=w553:bool)
                      n397 = Wait Until Next ms Multiple(millisecond multiple=u32 100 ("毫秒倍数")) -> ()  [unwired: 1 out]
                      n398 = Compound Arithmetic op=OR(w550, w551, w553) -> (w552:bool)
                    }
                  }
                  frame #4 {
                    n399 = case shown="假" w558 {
                      tunnel: w557 -> [w559 w565]
                      frame False {
                        n400 = control-ref of="结果"() -> (w563:refnum<vi>)
                        n401 = Concatenate Strings(w559, "       写入失败" ("字符串")) -> (w562:string)
                        n402 = Build Array(w562) -> (w561:string[])
                        n403 = call "表格编辑.vi"("新元素/子数组"=w561, "活动单元格:单元格背景色"=u32 16740749, "MCListbox引用句柄"=w563) -> ()  [unwired: 9 out]
                      }
                      frame True {
                        n404 = case shown="\"从板号\"" w565 {
                          frame "假", Default {
                          }
                          frame "从板号" {
                            n405 = local read "从板号"() -> (w566:u8)
                            n406 = local write "当前从板板号"(w566) -> ()
                          }
                        }
                      }
                    }
                    n407 = call <vilib>:"Unset Busy.vi"() -> ()  [unwired: 2 in, 10 out]
                  }
                  frame #5 {
                    n408 = Increment(x=w569) -> (x+1=w568:i32)
                    n409 = Equal?(x=w570, y=w568) -> (x = y?=w567:bool)
                    n410 = case shown="真" w567 {
                      frame False {
                      }
                      frame True {
                        n411 = control-ref of="结果"() -> (w574:refnum<vi>)
                        n412 = Concatenate Strings("写入完成" ("字符串")) -> (w573:string)
                        n413 = Build Array(w573) -> (w572:string[])
                        n414 = call "表格编辑.vi"("新元素/子数组"=w572, "活动单元格:单元格背景色"=u32 21937, "MCListbox引用句柄"=w574) -> ()  [unwired: 9 out]
                      }
                    }
                  }
                }
              }
            }
          }
          n415 = stacked-sequence {
            tunnel: w448 -> [_]
            frame #0 {
              n416 = call <vilib>:"Unset Busy.vi"() -> ()  [unwired: 2 in, 10 out]
              n417 = local write "强制终止读写标记"(FALSE ("强制停止")) -> ()
            }
          }
        }
        frame "全部写入" {
          n418 = local read "主从选择"() -> (w581:enum32{"主板", "从板"})
          n419 = case shown="\"主板\", 默认" w581 {
            tunnel: [string[] ["项目信息", "一级故障阀值", "二级故障阀值", "三级故障阀值", "加热控制参数", "充电控制参数", "电池信息"] string[] ["从板信息", "一级故障阀值", "二级故障阀值", "三级故障阀值", "均衡参数"]] -> w578
            tunnel: [0.0 ("从板号") w710] -> w582
            tunnel: [w695 _] -> w580
            tunnel: [_ w711] -> w579
            frame "主板", Default {
              n420 = stacked-sequence {
                tunnel: [_ w709] -> w695
                frame #0 {
                  n421 = control-ref of="电池信息"() -> (w701:refnum<vi>)
                  n422 = control-ref of="高压参数"() -> (w700:refnum<vi>)
                  n423 = control-ref of="一级故障"() -> (w703:refnum<vi>)
                  n424 = control-ref of="一级故障 2"() -> (w705:refnum<vi>)
                  n425 = control-ref of="一级故障 3"() -> (w706:refnum<vi>)
                  n426 = control-ref of="加热控制参数"() -> (w707:refnum<vi>)
                  n427 = control-ref of="充电控制参数"() -> (w708:refnum<vi>)
                  n428 = control-ref of="项目信息"() -> (w704:refnum<vi>)
                  n429 = control-ref of="项目信息2"() -> (w702:refnum<vi>)
                  n430 = local read "主板数据"() -> (w699:T4)
                  n431 = Bundle(cluster=w699, "项目信息"=w704, "一级故障 4"=w702, "一级故障"=w703, "一级故障 2"=w705, "一级故障 3"=w706, "加热控制参数"=w707, "充电控制参数"=w708, "高压参数"=w700, "电池信息"=w701) -> (w698:T4)
                  n432 = local write "主板数据"(w698) -> ()
                }
                frame #1 {
                  n433 = control-ref of="主板数据"() -> (w709:refnum<vi>)
                }
              }
            }
            frame "从板" {
              (unwired) "均衡参数"
              n434 = stacked-sequence {
                tunnel: [_ w723] -> w711
                frame #0 {
                  n435 = control-ref of="从板号"() -> (w717:refnum<vi>)
                  n436 = control-ref of="项目信息 2"() -> (w718:refnum<vi>)
                  n437 = control-ref of="均衡参数"() -> (w715:refnum<vi>)
                  n438 = control-ref of="加热控制参数"() -> (w719:refnum<vi>)
                  n439 = control-ref of="一级故障(从板)"() -> (w720:refnum<vi>)
                  n440 = control-ref of="二级故障(从板)"() -> (w721:refnum<vi>)
                  n441 = control-ref of="三级故障(从板)"() -> (w722:refnum<vi>)
                  n442 = control-ref of="电池组信息"() -> (w716:refnum<vi>)
                  n443 = local read "从板信息"() -> (w714:T2)
                  n444 = Bundle(cluster=w714, "从板号"=w717, "项目信息 2"=w718, "加热控制参数"=w719, "一级故障(从板)"=w720, "二级故障(从板)"=w721, "三级故障(从板)"=w722, "电池组信息(从板)"=w716, "均衡参数"=w715) -> (w713:T2)
                  n445 = local write "从板信息"(w713) -> ()
                }
                frame #1 {
                  n446 = control-ref of="从板信息"() -> (w723:refnum<vi>)
                }
              }
              n447 = local read "从板号"() -> (w710:u8)
            }
          }
          n448 = Array Size(array=w578) -> (size(s)=w577:i32)
          n449 = while {
            tunnel: w578 -> [w590] mode=indexing
            tunnel: w581 -> [w594]
            tunnel: w582 -> [w597]
            tunnel: w580 -> [w596]
            tunnel: w579 -> [w595]
            tunnel: w577 -> [w588]
            tunnel: [w584] -> w576
            i -> [w589]
            stop <- w585 stop-if-true
            n450 = Increment(x=w589) -> (x+1=w587:i32)
            n451 = local read "从板个数"() -> (w602:dbl)
            n452 = local read "快换"() -> (w593:bool)
            n453 = Less Or Equal?(x=w588, y=w587) -> (x <= y?=w584:bool)
            n454 = call "输入数据解析.vi"("单个参数补充"=w602, "从板号"=w597, "主板引用"=w596, "从板引用"=w595, "主板选项"=w590, "枚举"=w594, "快换"=w593) -> ("输出数组"=w601:dbl[][], "数组长度"=w600:dbl[], "循环次数"=w592:i32, "命令"=w599:u32, "名称"=w591:string[], "命令序号"=w598:u32[])  [unwired: 2 in, 1 out]
            n455 = case shown="\"主板\", 默认" w594 {
              tunnel: w589 -> [w604 w618]
              frame "主板", Default {
                n456 = case shown="6" w604 {
                  tunnel: [T8."项目信息" ("主从板") T8."一级故障阀值" ("主从板") T8."二级故障阀值" ("主从板") T8."三级故障阀值" ("主从板") T8."控制参数" ("主从板") T8."电池信息" ("主从板")] -> w603
                  frame 0, Default {
                    n457 = local write "1"(TRUE ("1")) -> ()
                  }
                  frame 1 {
                    n458 = local write "1 2"(TRUE ("1 2")) -> ()
                  }
                  frame 2 {
                    n459 = local write "1 3"(TRUE ("1 3")) -> ()
                  }
                  frame 3 {
                    n460 = local write "1 4"(TRUE ("1 4")) -> ()
                  }
                  frame 4, 5 {
                    n461 = local write "1 5"(TRUE ("1 5")) -> ()
                  }
                  frame 6 {
                    n462 = local write "1 11"(TRUE ("1 11")) -> ()
                  }
                }
                n463 = local write "主板2"(w603) -> ()
              }
              frame "从板" {
                n464 = case shown="1" w618 {
                  tunnel: [T19."从板信息" ("等级 2") T19."从板信息" ("等级 2") T19."一级故障阀值" ("等级 2") T19."二级故障阀值" ("等级 2") T19."三级故障阀值" ("等级 2") T19."快换参数" ("等级 2") T14."均衡参数" ("等级 2")] -> w617
                  frame 99, Default {
                    n465 = local write "1 6"(TRUE ("1 6")) -> ()
                  }
                  frame 0 {
                    n466 = local write "1 6"(TRUE ("1 6")) -> ()
                  }
                  frame 1 {
                    n467 = local write "1 7"(TRUE ("1 7")) -> ()
                  }
                  frame 2 {
                    n468 = local write "1 8"(TRUE ("1 8")) -> ()
                  }
                  frame 3 {
                    n469 = local write "1 9"(TRUE ("1 9")) -> ()
                  }
                  frame 4 {
                    n470 = local write "1 10"(TRUE ("1 10")) -> ()
                  }
                  frame 5 {
                    n471 = local write "1 12"(TRUE ("1 10")) -> ()
                  }
                }
                n472 = local write "等级 2"(w617) -> ()
              }
            }
            n473 = for {
              N: w592 -> [w635]
              tunnel: w601 -> [w645]
              tunnel: w600 -> [w644]
              tunnel: w599 -> [w643]
              tunnel: w598 -> [w641]
              tunnel: w597 -> [w642]
              tunnel: w591 -> [w638]
              tunnel: w584 -> [w633]
              i -> [w634]
              n474 = Index Array(array=w645, index (row)=w634) -> (element=w640:dbl[])  [unwired: 1 in]
              n475 = Index Array(array=w644, index=w634) -> (element=w639:dbl)
              n476 = Index Array(array=w638, index=w634) -> (element=w636:string)
              n477 = Index Array(array=w641, index=w634) -> (element=w637:u32)
              n478 = stacked-sequence {
                seq-local: [_ _ _ w668 _ _] -> [_ _ _ _ w677 _]
                tunnel: w640 -> [_ _ w656 _ _ _]
                tunnel: w639 -> [_ _ w655 _ _ _]
                tunnel: w643 -> [_ _ w650 _ _ _]
                tunnel: w642 -> [_ _ w653 _ _ _]
                tunnel: w637 -> [_ _ w651 _ _ _]
                tunnel: w636 -> [_ _ w649 _ w676 _]
                tunnel: w635 -> [_ _ _ _ _ w689]
                tunnel: w634 -> [_ _ _ _ _ w688]
                tunnel: w633 -> [_ _ _ _ _ w686]
                frame #0 {
                  w647 = FALSE ("流控帧")
                  w646 = TRUE ("流控帧 2")
                  n479 = call <vilib>:"Set Busy.vi"("disable click? (T)"=w647) -> ()  [unwired: 3 in, 8 out]
                  n480 = global write "EV05全局变量1.vi" "读取超时"(w647) -> ()
                  n481 = global write "EV05全局变量1.vi" "流控帧"(w647) -> ()
                  n482 = local write "消除"(w646) -> ()
                  n483 = local write "控制1"(w646) -> ()
                  n484 = global write "EV05全局变量1.vi" "流控帧 2"(w646) -> ()
                  n485 = local write "写?"(w646) -> ()
                }
                frame #1 {
                  n486 = Wait Until Next ms Multiple(millisecond multiple=u32 50 ("毫秒倍数")) -> ()  [unwired: 1 out]
                }
                frame #2 {
                  n487 = global write "全局 1.vi" "名称"(w649) -> ()
                  n488 = local write "命令序号"(w651) -> ()
                  n489 = local write "命令"(w650) -> ()
                  n490 = local read "设备索引号"() -> (w658:u16)
                  n491 = local read "CAN卡类型"() -> (w659:u32)
                  n492 = Increment(x=w655) -> (x+1=w652:dbl)
                  n493 = local read "CAN端口"() -> (w657:u16)
                  n494 = Reshape Array(w656, w652) -> (w654:dbl[])
                  n495 = stacked-sequence {
                    tunnel: w659 -> [_ w667]
                    tunnel: w658 -> [_ w666]
                    tunnel: w657 -> [_ w665]
                    tunnel: w654 -> [_ w664]
                    tunnel: w653 -> [_ w663]
                    tunnel: w651 -> [_ w662]
                    tunnel: w650 -> [_ w661]
                    frame #0 {
                    }
                    frame #1 {
                      n496 = call "多帧发送机制(EV05).vi"("can卡类型"=w667, "设备索引号"=w666, "CAN端口"=w665, "命令"=w661, "板号"=w663, "命令序号"=w662, "输入数据"=w664) -> ("错误输出"=w660:errorcluster)  [unwired: 2 in, 10 out]
                      n497 = call <vilib>:"Clear Errors.vi"("error in (no error)"=w660) -> ()  [unwired: 6 in, 1 out]
                    }
                  }
                }
                frame #3 {
                  n498 = while {
                    tunnel: [w670] -> w668
                    i -> [w675]
                    stop <- w672 stop-if-true
                    n499 = local read "强制终止读写标记"() -> (w669:bool)
                    n500 = global read "EV05全局变量1.vi" "读取超时"() -> (w670:bool)
